vi "test Multi FPGA Feature Toggle.vi"(8 "error in (no error)":errorcluster, 11 "TestCase in":refnum<class "Mutation Test Case.lvclass">) -> (0 "error out":errorcluster, 3 "TestCase out":refnum<class "Mutation Test Case.lvclass">)   [LabVIEW 2015, in "Mutation Test Case.lvclass"]
uses:
  Mutation Test Case.lvclass
  Shared/Properties.vi
  Shared/Constants and GUIDs.vi
  <vilib>/NI Veristand/Custom Device API/Get Item Property (String Array).vi
  <vilib>/NI Veristand/Custom Device Tools/Custom Device Utility Library/NI VeriStand - Search for All Items by GUID.vi
  <vilib>/NI Veristand/Custom Device API/Get Item Property (String).vi
  <vilib>/NI Veristand/Custom Device API/Get Item Property (Boolean).vi
  <vilib>/addons/_JKI Toolkits/VI Tester/TestCase.llb/TestCase.lvclass
  System Explorer/Engine Simulation Toolkit System Explorer.lvlib
  <vilib>/NI VeriStand/Custom Device API/Custom Device API.lvlib
  Shared/Engine Simulation Toolkit Shared.lvlib
  <vilib>/NI VeriStand/Custom Device Tools/Custom Device Utility Library/Custom Device Utility Library.lvlib
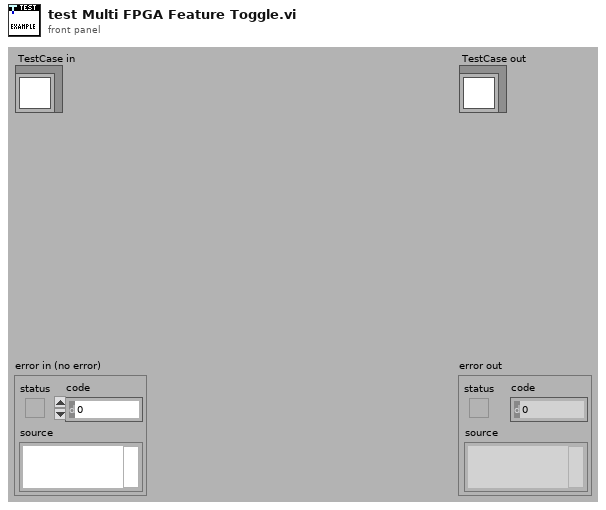
[diagram p1: front panel]
types:
  T1 = typedef "Custom Device API.lvlib/Custom Device Item Ref.ctl" = u64
  T2 = typedef "Custom Device API.lvlib/Custom Device Item Info.ctl" = cluster{"Name":string, "Is Channel":bool, "GUID":string, "Is Waveform":bool}
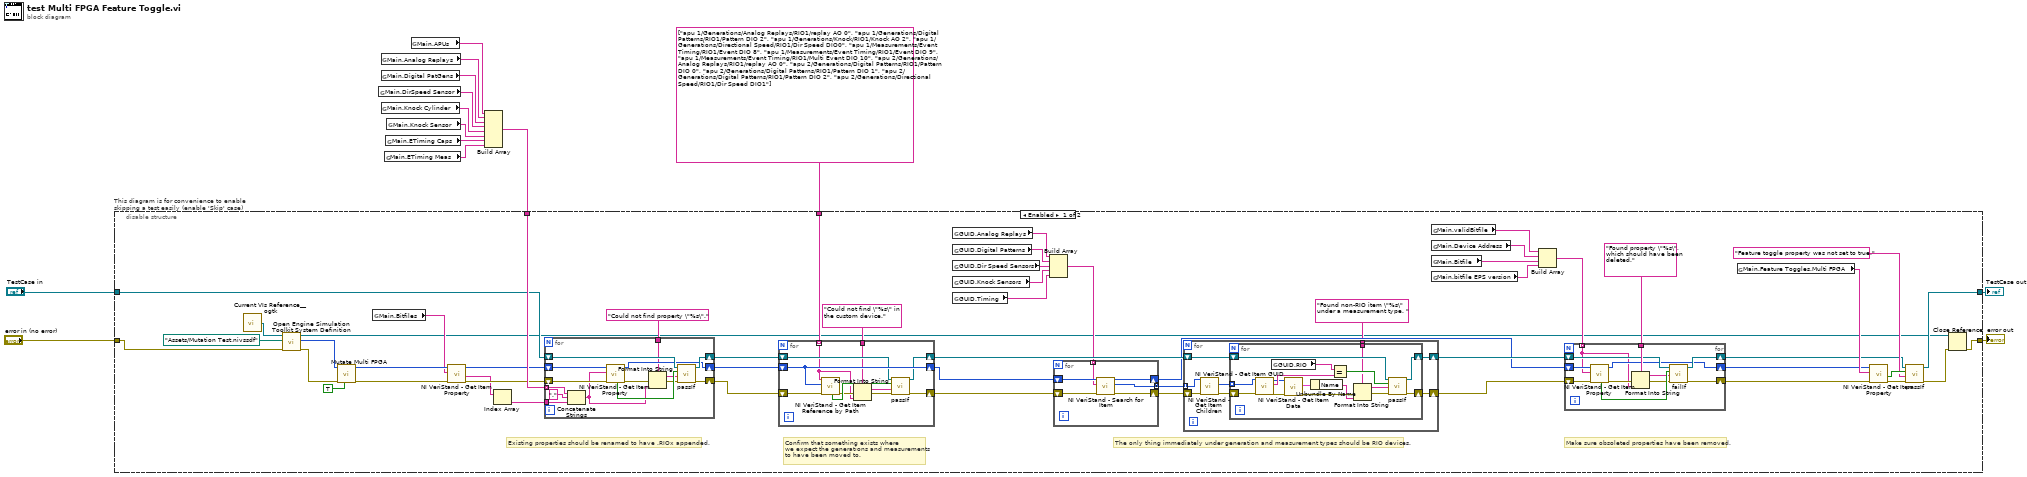
[diagram p0: block diagram]
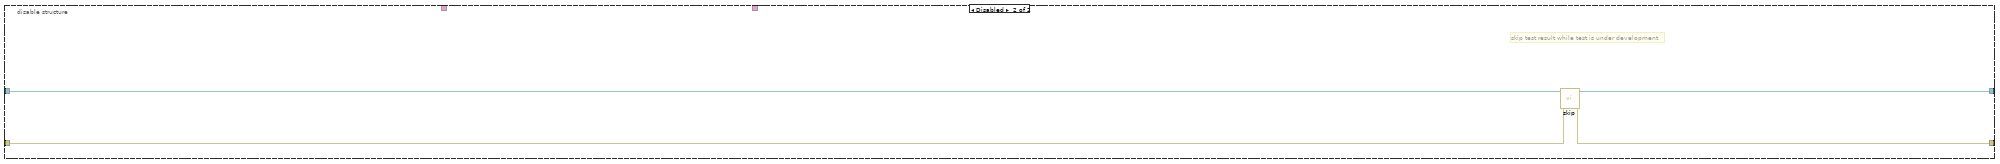
[diagram p2: hidden frame]
diagram:
  n1 = global read "Properties.vi" "Main.DirSpeed Sensor"() -> (w6:string)
  n2 = global read "Properties.vi" "Main.Analog Replays"() -> (w4:string)
  n3 = global read "Properties.vi" "Main.Digital PatGens"() -> (w5:string)
  n4 = global read "Properties.vi" "Main.Knock Cylinder"() -> (w7:string)
  n5 = global read "Properties.vi" "Main.ETiming Meas"() -> (w9:string)
  n6 = global read "Properties.vi" "Main.ETiming Caps"() -> (w8:string)
  n7 = global read "Properties.vi" "Main.Knock Sensor"() -> (w10:string)
  n8 = global read "Properties.vi" "Main.APUs"() -> (w3:string)
  n9 = Build Array(w3, w4, w5, w6, w7, w10, w8, w9) -> (w2:string[])
  n10 = disable-structure "This diagram is for convenience to enable skipping a test easily (enable 'Skip' case)" shown="Enabled" {
    disable-tunnel: "TestCase in" -> [w18 w139]
    disable-tunnel: [w53 w137] -> w12
    disable-tunnel: [w46 w138] -> w1
    disable-tunnel: "error in (no error)" -> [w65 w136]
    disable-tunnel: string[] ["apu 1/Generations/Analog Replays/RIO1/replay AO 0", "apu 1/Generations/Digital Patterns/RIO1/Pattern DIO 2", "apu 1/Generations/Knock/RIO1/Knock AO 2", "apu 1/Generations/Directional Speed/RIO1/Dir Speed DIO0", "apu 1/Measurements/Event Timing/RIO1/Event DIO 8", "apu 1/Measurements/Event Timing/RIO1/Event DIO 9", "apu 1/Measurements/Event Timing/RIO1/Multi Event DIO 10", "apu 2/Generations/Analog Replays/RIO1/replay AO 0", "apu 2/Generations/Digital Patterns/RIO1/Pattern DIO 0", "apu 2/Generations/Digital Patterns/RIO1/Pattern DIO 1", "apu 2/Generations/Digital Patterns/RIO1/Pattern DIO 2", "apu 2/Generations/Directional Speed/RIO1/Dir Speed DIO1"] ("string array") -> [w45 _]
    disable-tunnel: w2 -> [w26 _]
    frame Enabled {
      # "Existing properties should be renamed to have .RIOx appended."
      # "Make sure obsoleted properties have been removed."
      # "The only thing immediately under generation and measurement types should be RIO devices."
      # "Confirm that something exists where\nwe expect the generations and measurements\nto have been moved to."
      n11 = call <userlib>:"Current VIs Reference__ogtk.vi"() -> ("Current VI's reference"=w67:refnum<vi>)  [unwired: 5 in]
      n12 = call "Open Engine Simulation Toolkit System Definition.vi"("error in (no error)"=w65, "System Definition Path"=path "Assets/Mutation Test.nivssdf" ("Absolute or Relative Path"), "Current VI in"=w67) -> ("error out"=w48:errorcluster, "Engine Simulation Toolkit NodeID"=w64:u64, "SystemDefinition"=w16:refnum<k24>)  [unwired: 6 in]
      n13 = call "Mutate Multi FPGA.vi"("Force (F)"=TRUE, "error in (no error)"=w48, "Device Ref in"=w64) -> ("error out"=w15:errorcluster, "Device Ref out"=w25:T1)  [unwired: 7 in]
      n14 = global read "Properties.vi" "Main.Bitfiles"() -> (w22:string)
      n15 = call-poly <vilib>:"NI VeriStand - Get Item Property.vi"("error in (no error)"=w15, "Property Name"=w22, "Item Ref in"=w25) -> ("error out"=w24:errorcluster, "Value"=w21:string[], "Item Ref out"=w23:T1)  [unwired: 5 in, 1 out]
      n16 = Index Array(array=w21) -> (element=w20:string)  [unwired: 1 in]
      n17 = for {
        tunnel: w26 -> [w81] mode=indexing
        shift-right: [w77] -> w28
        shift-left: w24 -> [w79]
        shift-right: [w74] -> w27
        shift-left: w23 -> [w78]
        tunnel: w20 -> [w80]
        shift-right: [w75] -> w19
        shift-left: w18 -> [w76]
        tunnel: "Could not find property \"%s\"." ("format string") -> [w68]
        n18 = Concatenate Strings(w81, "." ("string"), w80) -> (w69:string)
        n19 = call-poly <vilib>:"NI VeriStand - Get Item Property.vi"("error in (no error)"=w79, "Property Name"=w69, "Item Ref in"=w78) -> ("error out"=w72:errorcluster, "Item Ref out"=w74:T1, "Found?"=w73:bool)  [unwired: 5 in, 1 out]
        n20 = Format Into String(format string=w68, error in=w72, w69) -> (resulting string=w70:string, error out=w71:errorcluster)  [unwired: 1 in]
        n21 = call-dynamic "passIf.vi"("error in (no error)"=w71, "message (\"\")"=w70, "pass"=w73, "TestCase in"=w76) -> ("error out"=w77:errorcluster, "TestCase out"=w75:refnum<class "Mutation Test Case.lvclass">)  [unwired: 6 in]
      }
      n22 = for {
        shift-right: [w90] -> w40
        shift-left: w28 -> [w92]
        shift-right: [w93] -> w37
        shift-left: w27 -> [w93]
        tunnel: w45 -> [w84] mode=indexing
        shift-right: [w88] -> w42
        shift-left: w19 -> [w89]
        tunnel: "Could not find \"%s\" in the custom device." ("format string") -> [w83]
        n23 = call <vilib>:"NI VeriStand - Get Item Reference by Path.vi"("error in (no error)"=w92, "Root Ref"=w93, "Item Path in"=w84) -> ("error out"=w87:errorcluster, "Found"=w91:bool)  [unwired: 5 in, 2 out]
        n24 = Format Into String(format string=w83, error in=w87, w84) -> (resulting string=w85:string, error out=w86:errorcluster)  [unwired: 1 in]
        n25 = call-dynamic "passIf.vi"("error in (no error)"=w86, "message (\"\")"=w85, "pass"=w91, "TestCase in"=w89) -> ("error out"=w90:errorcluster, "TestCase out"=w88:refnum<class "Mutation Test Case.lvclass">)  [unwired: 6 in]
      }
      n26 = global read "Constants and GUIDs.vi" "GUID.Analog Replays"() -> (w30:string)
      n27 = global read "Constants and GUIDs.vi" "GUID.Digital Patterns"() -> (w31:string)
      n28 = global read "Constants and GUIDs.vi" "GUID.Dir Speed Sensors"() -> (w32:string)
      n29 = global read "Constants and GUIDs.vi" "GUID.Knock Sensors"() -> (w33:string)
      n30 = global read "Constants and GUIDs.vi" "GUID.Timing"() -> (w34:string)
      n31 = Build Array(w30, w31, w32, w33, w34) -> (w29:string[])
      n32 = for {
        tunnel: [w97] -> w38 mode=concatenating
        shift-right: [w98] -> w39
        shift-left: w40 -> [w99]
        shift-right: [w95] -> w36
        shift-left: w37 -> [w96]
        tunnel: w29 -> [w94] mode=indexing
        n33 = call-poly <vilib>:"NI VeriStand - Search for Item.vi"("error in"=w99, "Item GUID"=w94, "Section Ref in"=w96) -> ("error out"=w98:errorcluster, "Item Refs"=w97:T1[], "Section Ref out"=w95:T1)  [unwired: 5 in, 1 out]
      }
      n34 = for {
        shift-right: [w105] -> w41
        shift-left: w42 -> [w104]
        shift-right: [w103] -> w43
        shift-left: w39 -> [w102]
        tunnel: w38 -> [w101] mode=indexing
        tunnel: "Found non-RIO item \"%s\" under a measurement type. " ("format string") -> [w100]
        n35 = call <vilib>:"NI VeriStand - Get Item Children.vi"("error in (no error)"=w102, "Item Ref in"=w101) -> ("error out"=w107:errorcluster, "Child Refs"=w106:T1[])  [unwired: 6 in, 2 out]
        n36 = for {
          shift-right: [w123] -> w103
          shift-left: w107 -> [w121]
          tunnel: w106 -> [w119] mode=indexing
          shift-right: [w118] -> w105
          shift-left: w104 -> [w117]
          tunnel: w100 -> [w113]
          n37 = call <vilib>:"NI VeriStand - Get Item GUID.vi"("error in (no error)"=w121, "Item Ref in"=w119) -> ("error out"=w112:errorcluster, "GUID"=w122:string, "Item Ref out"=w111:T1)  [unwired: 7 in]
          n38 = global read "Constants and GUIDs.vi" "GUID.RIO"() -> (w116:string)
          n39 = call <vilib>:"NI VeriStand - Get Item Data.vi"("error in (no error)"=w112, "Item Ref in"=w111) -> ("error out"=w109:errorcluster, "Item Info"=w110:T2)  [unwired: 6 in, 2 out]
          n40 = Unbundle By Name(w110) -> ("Name"=w108:string)
          n41 = Equal?(x=w116, y=w122) -> (x = y?=w120:bool)
          n42 = Format Into String(format string=w113, error in=w109, w108) -> (resulting string=w114:string, error out=w115:errorcluster)  [unwired: 1 in]
          n43 = call-dynamic "passIf.vi"("error in (no error)"=w115, "message (\"\")"=w114, "pass"=w120, "TestCase in"=w117) -> ("error out"=w123:errorcluster, "TestCase out"=w118:refnum<class "Mutation Test Case.lvclass">)  [unwired: 6 in]
        }
      }
      n44 = global read "Properties.vi" "Main.validBitfile"() -> (w61:string)
      n45 = global read "Properties.vi" "Main.Device Address"() -> (w62:string)
      n46 = global read "Properties.vi" "Main.Bitfile"() -> (w60:string)
      n47 = global read "Properties.vi" "Main.bitfile EPS version"() -> (w59:string)
      n48 = Build Array(w61, w62, w60, w59) -> (w58:string[])
      n49 = for {
        shift-right: [w131] -> w55
        shift-left: w43 -> [w134]
        shift-right: [w132] -> w49
        shift-left: w41 -> [w129]
        tunnel: w58 -> [w124] mode=indexing
        tunnel: "Found property \"%s\", which should have been deleted." ("format string") -> [w130]
        shift-right: [w125] -> w54
        shift-left: w36 -> [w135]
        n50 = call-poly <vilib>:"NI VeriStand - Get Item Property.vi"("error in (no error)"=w134, "Property Name"=w124, "Item Ref in"=w135) -> ("error out"=w128:errorcluster, "Item Ref out"=w125:T1, "Found?"=w133:bool)  [unwired: 5 in, 1 out]
        n51 = Format Into String(format string=w130, error in=w128, w124) -> (resulting string=w126:string, error out=w127:errorcluster)  [unwired: 1 in]
        n52 = call-dynamic "failIf.vi"("error in (no error)"=w127, "message (\"\")"=w126, "fail"=w133, "TestCase in"=w129) -> ("error out"=w131:errorcluster, "TestCase out"=w132:refnum<class "Mutation Test Case.lvclass">)  [unwired: 6 in]
      }
      n53 = global read "Properties.vi" "Main.Feature Toggles.Multi FPGA"() -> (w56:string)
      n54 = call-poly <vilib>:"NI VeriStand - Get Item Property.vi"("error in (no error)"=w55, "Property Name"=w56, "Item Ref in"=w54) -> ("error out"=w52:errorcluster, "Value"=w51:bool)  [unwired: 5 in, 2 out]
      n55 = call-dynamic "passIf.vi"("error in (no error)"=w52, "message (\"\")"="Feature toggle property was not set to true." ("message (\"\")"), "pass"=w51, "TestCase in"=w49) -> ("error out"=w47:errorcluster, "TestCase out"=w53:refnum<class "Mutation Test Case.lvclass">)  [unwired: 6 in]
      n56 = Close Reference(reference=w16, error in (no error)=w47) -> (error out=w46:errorcluster)
    }
    frame Disabled {
      # "skip test result while test is under development"
      n57 = call <vilib>:"skip.vi"("error in (no error)"=w136, "TestCase in"=w139) -> ("error out"=w138:errorcluster, "TestCase out"=w137:refnum<class "Mutation Test Case.lvclass">)  [unwired: 8 in]
    }
  }
  "error out" <- w1
  "TestCase out" <- w12
